vi "Launcher.vi"() -> ()   [LabVIEW 2014, in "Camera Actor.lvlib"]
uses:
  Camera Actor.lvlib
  Camera Actor/Camera Actor.lvclass
  <vilib>/userdefined/High Color/IMAQdx.ctl
  Camera Actor Messages/Start Acquisition Msg/Start Acquisition Msg.lvclass/Start Acquisition Msg.ctl
  <vilib>/ActorFramework/Message Enqueuer/Message Enqueuer.lvclass/Message Enqueuer.ctl
  <vilib>/ActorFramework/Message Enqueuer/Message Priority.ctl
  <vilib>/ActorFramework/Message Enqueuer/Enqueue.vi
  <vilib>/ActorFramework/Message Priority Queue/Priority Enqueue.vi
  Camera Actor Messages/Start Acquisition Msg/Start Acquisition Msg.lvclass
  Camera Actor Messages/Stop Acquisition Msg/Stop Acquisition Msg.lvclass
  <vilib>/ActorFramework/Stop Msg/Stop Msg.lvclass
  Camera Actor Messages/open camera settings Msg/open camera settings Msg.lvclass
  <vilib>/ActorFramework/Actor/Actor.lvclass
  <vilib>/ActorFramework/Message Enqueuer/Message Enqueuer.lvclass
panel:
  in  "Settings":bool
  out "error out":errorcluster
  in  "Stop":bool
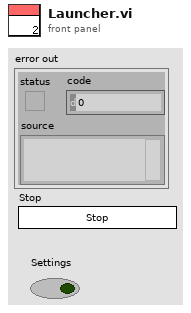
[diagram p1: front panel]
types:
  T1 = typedef "IMAQdx.ctl" = refnum<k21>
  T2 = typedef "Actor Framework.lvlib/Message Enqueuer.lvclass/Message Priority.ctl" = enum16{"Low", "Normal", "High"}
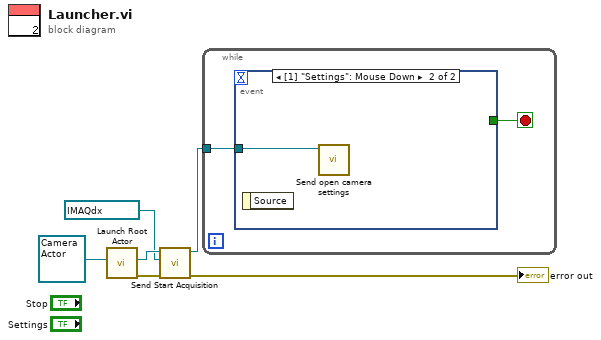
[diagram p0: block diagram]
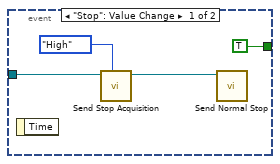
[diagram p2: hidden frame]
diagram:
  n1 = call <vilib>:"Launch Root Actor.vi"("Actor"=refnum<class "Camera Actor.lvclass"> refnum ("IMAQdx Actor.lvlib:IMAQdx Actor.lvclass")) -> ("error out"=w2:errorcluster, "Actor's Enqueuer"=w5:refnum<class "Message Enqueuer.lvclass">)  [unwired: 9 in]
  n2 = call "Send Start Acquisition.vi"("error in (no error)"=w2, "Camera Name"=T1 "TestCam", "Message Enqueuer"=w5) -> ("error out"=→"error out":errorcluster, "Message Enqueuer out"=w3:refnum<class "Message Enqueuer.lvclass">)  [unwired: 7 in]
  n3 = while {
    tunnel: w3 -> [w8]
    stop <- w7 stop-if-true
    n4 = event shown="[1] \"Settings\": Mouse Down" {
      selector: _ -> [_ _]
      dyn-events: _ -> [_ _]
      timeout: _ -> [_ _]
      tunnel: w8 -> [w11 w13]
      tunnel: [TRUE _] -> w7
      event "Stop": Value Change {
        n5 = event-data() -> ()  [unwired: 1 in, 1 out]
        n6 = call "Send Stop Acquisition.vi"("Message Priority (Normal)"=Message_Priority."High", "Message Enqueuer"=w11) -> ("Message Enqueuer out"=w10:refnum<class "Message Enqueuer.lvclass">)  [unwired: 8 in, 1 out]
        n7 = call <vilib>:"Send Normal Stop.vi"("Message Enqueuer"=w10) -> ()  [unwired: 10 in, 1 out]
      }
      event "Settings": Mouse Down {
        n8 = event-data() -> ()  [unwired: 1 in, 1 out]
        n9 = call "Send open camera settings.vi"("Message Enqueuer"=w13) -> ()  [unwired: 9 in, 2 out]
      }
    }
  }
